vi "Format SQL INSERT Dictionary.vi"(8 "error in (no error)":errorcluster, 10 "Data (Dictionary)":T1[](array[typedef]), 11 "table name":string) -> (0 "error out":errorcluster, 2 "SQL":string)   [LabVIEW 2016, in "LV-Data.PGSQL.lvclass"]
uses:
  LV-Data.PGSQL.lvclass
  LV-Data/Typedefs/Dictionary--cluster.ctl
  LV-Data/LV-Data.lvclass
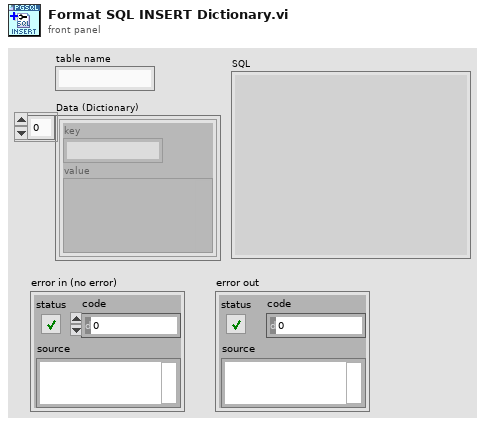
[diagram p1: front panel]
types:
  T1 = typedef "LV-Data.lvclass/Dictionary--cluster.ctl" = cluster{"key":string, "value":variant}
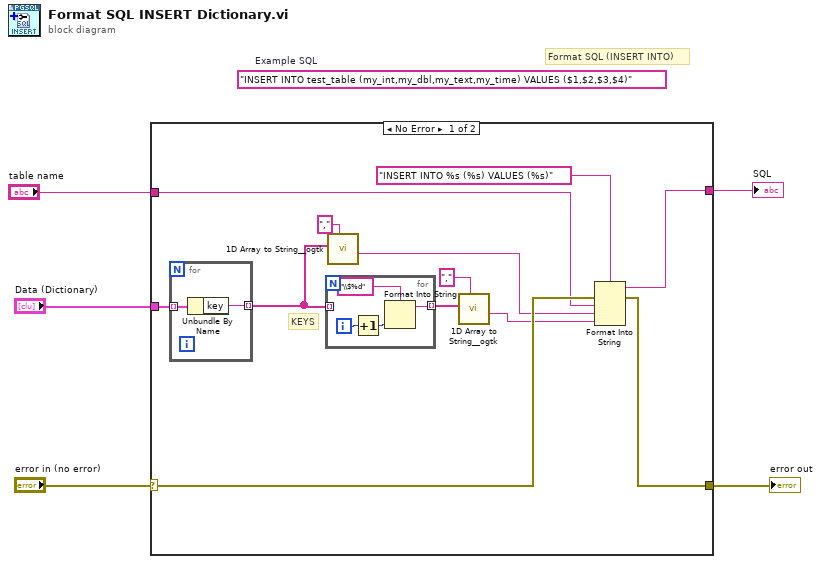
[diagram p0: block diagram]
diagram:
  (unwired) "INSERT INTO test_table (my_int,my_dbl,my_text,my_time) VALUES ($1,$2,$3,$4)"  # Example SQL
  # "Format SQL (INSERT INTO)"
  n1 = case shown="No Error" "error in (no error)" {
    selector: "error in (no error)" -> [w11 w24]
    tunnel: "Data (Dictionary)" -> [w7 _]
    tunnel: [w17 w24] -> w4
    tunnel: [w12 _] -> w3
    tunnel: "table name" -> [w10 _]
    frame No Error {
      # "KEYS"
      n2 = for {
        tunnel: w7 -> [w19] mode=indexing
        tunnel: [w18] -> w6 mode=indexing
        n3 = Unbundle By Name(w19) -> ("key"=w18:string)
      }
      n4 = for {
        tunnel: w6 -> [_] mode=indexing
        tunnel: [w21] -> w15 mode=indexing
        i -> [w23]
        n5 = Increment(x=w23) -> (x+1=w20:i32)
        n6 = Format Into String(format string="\\$%d", w20) -> (resulting string=w21:string)  [unwired: 2 in, 1 out]
      }
      n7 = call <userlib>:"1D Array to String__ogtk.vi"("delimiter (Tab)"=",", "Array of Strings"=w6) -> ("delimited string"=w9:string)  [unwired: 9 in]
      n8 = call <userlib>:"1D Array to String__ogtk.vi"("delimiter (Tab)"=",", "Array of Strings"=w15) -> ("delimited string"=w8:string)  [unwired: 9 in]
      n9 = Format Into String(format string="INSERT INTO %s (%s) VALUES (%s)" ("command"), error in=w11, w10, w9, w8) -> (resulting string=w12:string, error out=w17:errorcluster)  [unwired: 1 in]
    }
    frame Error {
    }
  }
  "SQL" <- w3
  "error out" <- w4
